vi "FOUR_U8_TO_FLOAT-1.vi"(1 "接收数据4*U8":u8[](array[numeric])) -> (0 "输出变量":dbl)   [LabVIEW 2018]
panel:
  # "四个字节高八位为整数位 低八位为小数位 经过转化为浮点数"
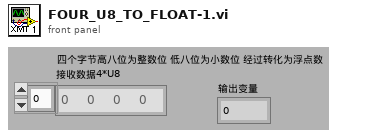
[diagram p1: front panel]
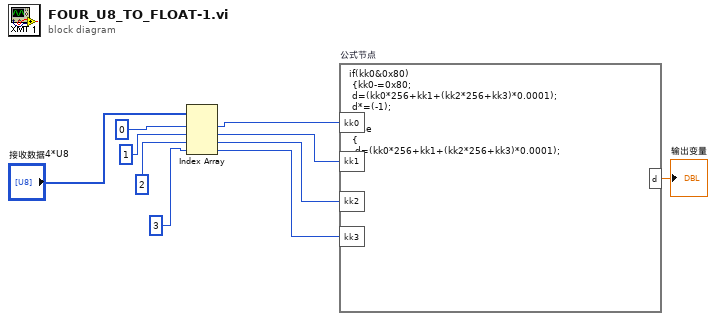
[diagram p0: block diagram]
diagram:
  n1 = Index Array(array="接收数据4*U8", index #1=0, index #2=1, index #3=2, index #4=3) -> (element #1=w5:u8, element #2=w4:u8, element #3=w3:u8, element #4=w2:u8)
  n2 = formula code="if(kk0&0x80)\n\t{kk0-=0x80;\n\td=(kk0*256+kk1+(kk2*256+kk3)*0.0001);\n\td*=(-1);\n\t}\n else\n\t{\n\t\td=(kk0*256+kk1+(kk2*256+kk3)*0.0001); \n}" "公式节点"("kk0"=w5, "kk1"=w4, "kk2"=w3, "kk3"=w2) -> ("d"=→"输出变量":dbl)
